vi "Main.vi"() -> ()   [LabVIEW 2018]
uses:
  Rectangle/Rectangle.lvclass/Rectangle.ctl
  Square/Square.lvclass
  C:/Users/plkruczp/National Instruments/IES Software Training Initiative - Documents/Software Design/LV Code/LSP/Rectangle/Rectangle.lvclass
  Rectangle/Rectangle.lvclass
panel:
  out "Everything OK":bool[](array[boolean])
  out "Violation of Contract":bool[](array[boolean])
  out "Square Area":dbl
  out "Rectangle Area":dbl
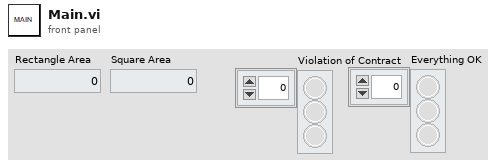
[diagram p1: front panel]
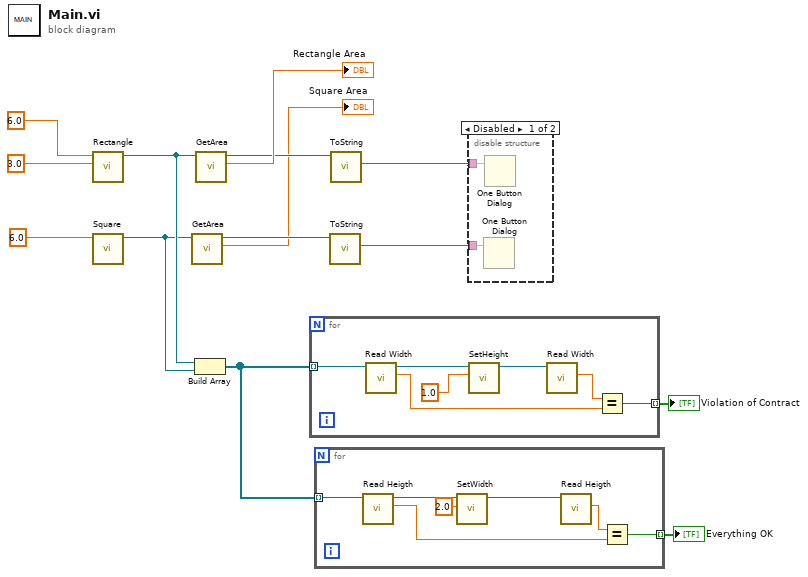
[diagram p0: block diagram]
diagram:
  n1 = call "Rectangle.vi"("Heigth"=3.0 ("Width"), "Width"=6.0) -> ("Rectangle Out"=w5:refnum<class "Rectangle.lvclass">)  [unwired: 9 in]
  n2 = call "Square.vi"("Side"=6.0) -> ("Square Out"=w4:refnum<class "Square.lvclass">)  [unwired: 10 in]
  n3 = call "GetArea.vi"("Rectangle In"=w4) -> ("Area"=→"Square Area":dbl, "Rectangle Out"=w7:refnum<class "Square.lvclass">)  [unwired: 9 in]
  n4 = Build Array(w5, w4) -> (w1:refnum<class "Rectangle.lvclass">[])
  n5 = call "GetArea.vi"("Rectangle In"=w5) -> ("Area"=→"Rectangle Area":dbl, "Rectangle Out"=w11:refnum<class "Rectangle.lvclass">)  [unwired: 9 in]
  n6 = for {
    tunnel: w1 -> [w19] mode=indexing
    tunnel: [w15] -> w3 mode=indexing
    n7 = call "Read Width.vi"("Rectangle in"=w19) -> ("Width"=w16:dbl, "Rectangle out"=w18:refnum<class "Rectangle.lvclass">)  [unwired: 9 in]
    n8 = call-dynamic "SetHeight.vi"("Height"=1.0 ("Width"), "Rectangle In"=w18) -> ("Rectangle Out"=w20:refnum<class "Rectangle.lvclass">)  [unwired: 9 in]
    n9 = call "Read Width.vi"("Rectangle in"=w20) -> ("Width"=w17:dbl)  [unwired: 9 in, 1 out]
    n10 = Equal?(x=w17, y=w16) -> (x = y?=w15:bool)
  }
  "Violation of Contract" <- w3
  n11 = for {
    tunnel: w1 -> [w26] mode=indexing
    tunnel: [w28] -> w2 mode=indexing
    n12 = call "Read Heigth.vi"("Rectangle in"=w26) -> ("Heigth"=w23:dbl, "Rectangle out"=w27:refnum<class "Rectangle.lvclass">)  [unwired: 9 in]
    n13 = call-dynamic "SetWidth.vi"("Width"=2.0, "Rectangle In"=w27) -> ("Rectangle Out"=w25:refnum<class "Rectangle.lvclass">)  [unwired: 9 in]
    n14 = call "Read Heigth.vi"("Rectangle in"=w25) -> ("Heigth"=w24:dbl)  [unwired: 9 in, 1 out]
    n15 = Equal?(x=w24, y=w23) -> (x = y?=w28:bool)
  }
  "Everything OK" <- w2
  n16 = call "ToString.vi"("Rectangle In"=w7) -> ("String"=w8:string)  [unwired: 9 in, 1 out]
  n17 = call "ToString.vi"("Rectangle In"=w11) -> ("String"=w10:string)  [unwired: 9 in, 1 out]
  n18 = disable-structure shown="Disabled" {
    disable-tunnel: w10 -> [w30 _]
    disable-tunnel: w8 -> [w29 _]
    frame Disabled {
      n19 = One Button Dialog(message=w29) -> ()  [unwired: 1 in, 1 out]
      n20 = One Button Dialog(message=w30) -> ()  [unwired: 1 in, 1 out]
    }
    frame Enabled {
    }
  }
